vi "Auto Recock Winch Half.vi"(11 "Run?":bool) -> (3 "Done":bool)   [LabVIEW 2013]
uses:
  Globals/Homes.vi
  <vilib>/addons/control/pid/pid.llb/PID (DBL).vi
  <vilib>/addons/control/pid/NI_PID_pid.lvlib
panel:
  in  "PID gains":T1={"proportional gain (Kc)"=2.75, "integral time (Ti, min)"=0.0, "derivative time (Td, min)"=0.0} {"derivative time (Td, min)" format="%.3f"; "integral time (Ti, min)" format="%.3f"; "proportional gain (Kc)" format="%.3f"}
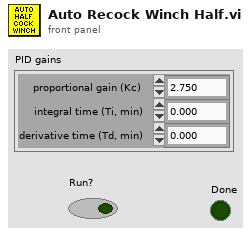
[diagram p1: front panel]
types:
  T1 = cluster{"proportional gain (Kc)":dbl, "integral time (Ti, min)":dbl, "derivative time (Td, min)":dbl}
  T2 = typedef "WPI_MotorControlDeviceRef.ctl" = cluster{"DeviceStatus":errorcluster, "Type":enum16{"PWM", "CAN"}, "PWM":cluster{"Digital Module":T3, "PWM Channel":T4, "DeadBand":T5}, "CAN":cluster{"Device Number":u8, "Control Mode":T6, "Semaphore":T7, "Max Vout":dbl}, "Invert":bool, "TransformRef":T8, "InvTransformRef":T8}
  T3 = typedef "FPGA_TypedefDigitalModule.ctl" = enum16{"Digital Module 1", "Digital Module 2"}
  T4 = typedef "FPGA_DIOPWMChannel.ctl" = enum8{"PWM 1", "PWM 2", "PWM 3", "PWM 4", "PWM 5", "PWM 6", "PWM 7", "PWM 8", "PWM 9", "PWM 10", "Invalid"}
  T5 = typedef "WPI_PWMDeadband.ctl" = cluster{"Name":string, "maxPositivePwm":i32, "minPositivePwm":i32, "centerPwm":i32, "maxNegativePwm":i32, "minNegativePwm":i32, "angularRange":u16}
  T6 = typedef "WPI_CANJaguar_ControlMode.ctl" = enum8{"Percent VBus", "Current", "Speed", "Position", "Voltage"}
  T7 = typedef "Semaphore RefNum" = refnum<k1>
  T8 = typedef "WPI_PWMTransform_ConPane.ctl" = refnum<vi>
  T9 = typedef "WPI_AnalogChannelDevRef.ctl" = cluster{"DevStatus":errorcluster, "Analog Module":T10, "Analog Channel":T11}
  T10 = typedef "FPGA_TypedefAnalogModule.ctl" = enum16{"Analog Module 1", "Analog Module 2"}
  T11 = typedef "FPGA_AIChannel.ctl" = enum8{"AI 1", "AI 2", "AI 3", "AI 4", "AI 5", "AI 6", "AI 7", "AI 8", "Invalid"}
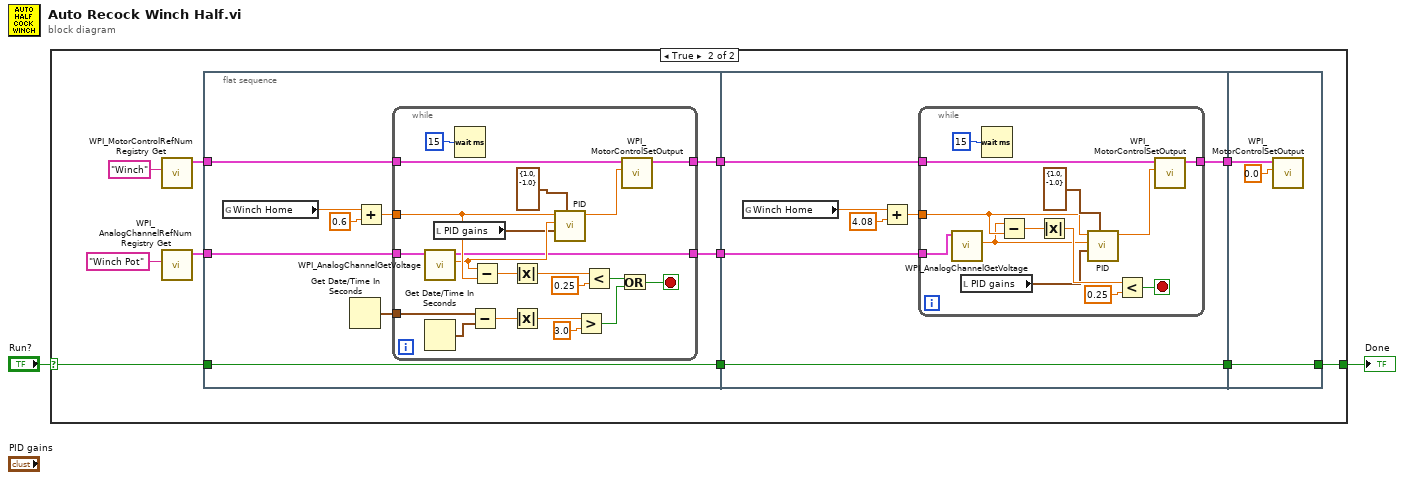
[diagram p0: block diagram]
diagram:
  n1 = case shown="True" "Run?" {
    selector: "Run?" -> [w3 w9]
    tunnel: [w3 w6] -> w1
    frame False {
    }
    frame True {
      n2 = call <vilib>:"WPI_MotorControlRefNum Registry Get.vi"("refnum name"="Winch") -> ("MotorControlDevRef"=w12:T2)  [unwired: 9 in, 1 out]
      n3 = call <vilib>:"WPI_AnalogChannelRefNum Registry Get.vi"("refnum name"="Winch Pot") -> ("AIDeviceRef"=w13:T9)  [unwired: 9 in, 1 out]
      n4 = flat-sequence {
        tunnel: w12 -> [w17]
        tunnel: w13 -> [w18]
        tunnel: w9 -> [w23]
        tunnel: [w23] -> w8
        tunnel: [w16] -> w5
        tunnel: [w15] -> w4
        tunnel: [w49] -> w14
        tunnel: [w48] -> w7
        tunnel: w4 -> [w50]
        tunnel: w5 -> [w47]
        tunnel: w8 -> [w48]
        tunnel: w14 -> [w67]
        tunnel: w7 -> [w65]
        tunnel: [w65] -> w6
        frame #0 {
          n5 = global read "Homes.vi" "Winch Home"() -> (w19:dbl)
          n6 = Get Date/Time In Seconds() -> (seconds since 1Jan1904=w22:timestamp)
          n7 = Add(x=w19, y=0.6) -> (x+y=w21:dbl)
          n8 = while {
            tunnel: w17 -> [w44]
            tunnel: w21 -> [w38]
            tunnel: w18 -> [w40]
            tunnel: [w36] -> w16
            tunnel: [w32] -> w15
            tunnel: w22 -> [w27]
            stop <- w25 stop-if-true
            n9 = call <vilib>:"WPI_AnalogChannelGetVoltage.vi"("AIDeviceRef"=w40) -> ("Voltage"=w37:dbl, "AIDeviceRef"=w32:T9)  [unwired: 8 in, 1 out]
            n10 = Get Date/Time In Seconds() -> (seconds since 1Jan1904=w28:timestamp)
            n11 = local read "PID gains"() -> (w35:T1)
            n12 = Wait (ms)(milliseconds to wait=u32 15) -> ()  [unwired: 1 out]
            n13 = Subtract(x=w27, y=w28) -> (x-y=w29:dbl)
            n14 = Subtract(x=w37, y=w38) -> (x-y=w43:dbl)
            n15 = Absolute Value(x=w43) -> (abs(x)=w42:dbl)
            n16 = Absolute Value(x=w29) -> (abs(x)=w30:dbl)
            n17 = call-poly <vilib>:"PID.vi"("output range"=cluster{"output high":dbl, "output low":dbl} {"output high"=1.0, "output low"=-1.0}, "PID gains"=w35, "process variable"=w37, "setpoint"=w38) -> ("output"=w33:dbl)  [unwired: 6 in, 1 out]
            n18 = Greater?(x=w30, y=3.0) -> (0:w26:bool)
            n19 = Less?(x=w42, y=0.25) -> (x < y?=w24:bool)
            n20 = Or(x=w24, y=w26) -> (x .or. y?=w25:bool)
            n21 = call <vilib>:"WPI_MotorControlSetOutput.vi"("Output"=w33, "MotorControlDevRef"=w44) -> ("MotorControlDevRef"=w36:T2)  [unwired: 7 in, 2 out]
          }
        }
        frame #1 {
          n22 = global read "Homes.vi" "Winch Home"() -> (w46:dbl)
          n23 = Add(x=w46, y=4.08) -> (x+y=w51:dbl)
          n24 = while {
            tunnel: w51 -> [w58]
            tunnel: w50 -> [w60]
            tunnel: [w56] -> w49
            tunnel: w47 -> [w53]
            stop <- w62 stop-if-true
            n25 = call <vilib>:"WPI_AnalogChannelGetVoltage.vi"("AIDeviceRef"=w60) -> ("Voltage"=w57:dbl)  [unwired: 8 in, 2 out]
            n26 = local read "PID gains"() -> (w52:T1)
            n27 = Wait (ms)(milliseconds to wait=u32 15) -> ()  [unwired: 1 out]
            n28 = Subtract(x=w57, y=w58) -> (x-y=w64:dbl)
            n29 = Absolute Value(x=w64) -> (abs(x)=w63:dbl)
            n30 = call-poly <vilib>:"PID.vi"("output range"=cluster{"output high":dbl, "output low":dbl} {"output high"=1.0, "output low"=-1.0}, "PID gains"=w52, "process variable"=w57, "setpoint"=w58) -> ("output"=w54:dbl)  [unwired: 6 in, 1 out]
            n31 = Less?(x=w63, y=0.25) -> (x < y?=w62:bool)
            n32 = call <vilib>:"WPI_MotorControlSetOutput.vi"("Output"=w54, "MotorControlDevRef"=w53) -> ("MotorControlDevRef"=w56:T2)  [unwired: 7 in, 2 out]
          }
        }
        frame #2 {
          n33 = call <vilib>:"WPI_MotorControlSetOutput.vi"("Output"=0.0, "MotorControlDevRef"=w67) -> ()  [unwired: 7 in, 3 out]
        }
      }
    }
  }
  "Done" <- w1
